vi "File Increment Logic.vi"(10 "error in (no error)":errorcluster, 11 "file name in":string) -> (2 "error out":errorcluster, 3 "file name out":string)   [LabVIEW 2025]
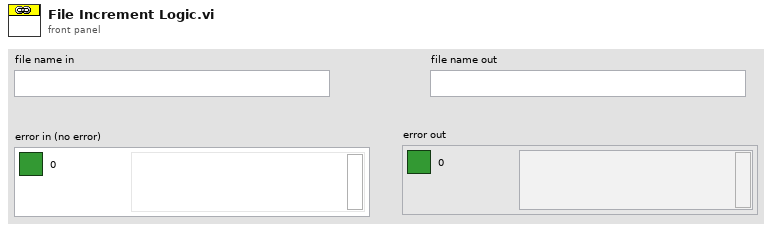
[diagram p1: front panel]
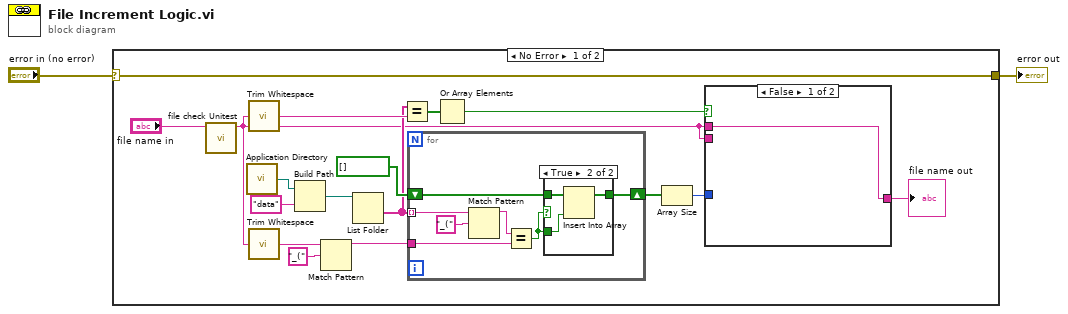
[diagram p0: block diagram]
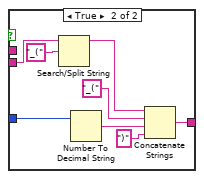
[diagram p2: hidden frame]
diagram:
  n1 = case shown="No Error" "error in (no error)" {
    selector: "error in (no error)" -> [w3 _]
    tunnel: [w3 _] -> w1
    frame No Error {
      n2 = call "file check Unitest.vi"("file name in"="file name in") -> ("file name out"=w6:string)  [unwired: 9 in, 1 out]
      n3 = call <vilib>:"Application Directory.vi"() -> ("Application Directory"=w16:path)
      n4 = call <vilib>:"Trim Whitespace.vi"("string"=w6) -> ("trimmed string"=w10:string)  [unwired: 1 in]
      n5 = call <vilib>:"Trim Whitespace.vi"("string"=w6) -> ("trimmed string"=w13:string)  [unwired: 1 in]
      n6 = Build Path(base path=w16, name or relative path="data") -> (appended path=w17:path)
      n7 = Match Pattern(string=w13, regular expression="_(") -> (before substring=w11:string)  [unwired: 1 in, 3 out]
      n8 = List Folder(path=w17) -> (folder names=w9:string[])  [unwired: 3 in, 3 out]
      n9 = Equal?(x=w9, y=w10) -> (x = y?=w12:bool[])
      n10 = for {
        tunnel: w9 -> [w34] mode=indexing
        tunnel: w11 -> [w32]
        shift-right: [w30] -> w19
        shift-left: bool[] [] -> [w31]
        n11 = Match Pattern(string=w34, regular expression="_(") -> (before substring=w33:string)  [unwired: 1 in, 3 out]
        n12 = Equal?(x=w33, y=w32) -> (x = y?=w29:bool)
        n13 = case shown="True" w29 {
          tunnel: w29 -> [_ w37]
          tunnel: w31 -> [w36 w39]
          tunnel: [w36 w38] -> w30
          frame False {
          }
          frame True {
            n14 = Insert Into Array(array=w39, new element=w37) -> (w38:bool[])  [unwired: 1 in]
          }
        }
      }
      n15 = Or Array Elements(Boolean array=w12) -> (logical OR=w8:bool)
      n16 = Array Size(array=w19) -> (size(s)=w7:i32)
      n17 = case shown="False" w8 {
        tunnel: w6 -> [_ w28]
        tunnel: w7 -> [_ w22]
        tunnel: [w20 w21] -> w4
        tunnel: w6 -> [w20 _]
        frame False {
        }
        frame True {
          n18 = Search/Split String(string=w28, search string/char (-)="_(" ("regular expression")) -> (substring before match=w26:string)  [unwired: 1 in, 2 out]
          n19 = Number To Decimal String(number=w22) -> (decimal integer string=w24:string)  [unwired: 1 in]
          n20 = Concatenate Strings(w26, "_(" ("regular expression"), w24, ")" ("regular expression")) -> (w21:string)
        }
      }
      "file name out" <- w4
    }
    frame Error {
    }
  }
  "error out" <- w1
